vi "Cross-corelation.vi"() -> ()   [LabVIEW 2017]
uses:
  <vilib>/Analysis/1siggen.llb/General Gaussian Monopulse.vi
  <vilib>/Analysis/2dsp.llb/1D Cross Correlation (DBL).vi
  <vilib>/Analysis/NI_AALPro.lvlib
  <vilib>/Analysis/NI_AAL_SigProc.lvlib
  <vilib>/Analysis/NI_AALBase.lvlib
panel:
  in  "Number of samples to \nshift second signal":i32=11
  out "Waveforms":dbl[][](graph)
  out "Sample Delay":dbl
  out "Cross Corelation":dbl[](graph)
  # "Overview: This example uses cross correlation to determine the sample delay between two signals that are identical but have been shifted.\nRequirements: LabVIEW 2012 ( or compatible)\nInstructions: \n1. Input the configuration in the control\n2. Run the VI"
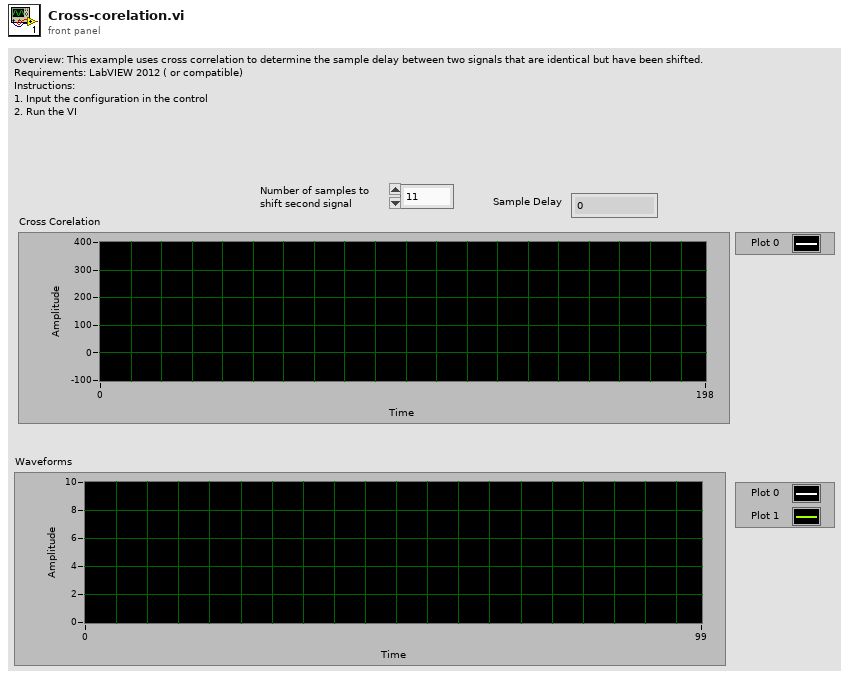
[diagram p1: front panel]
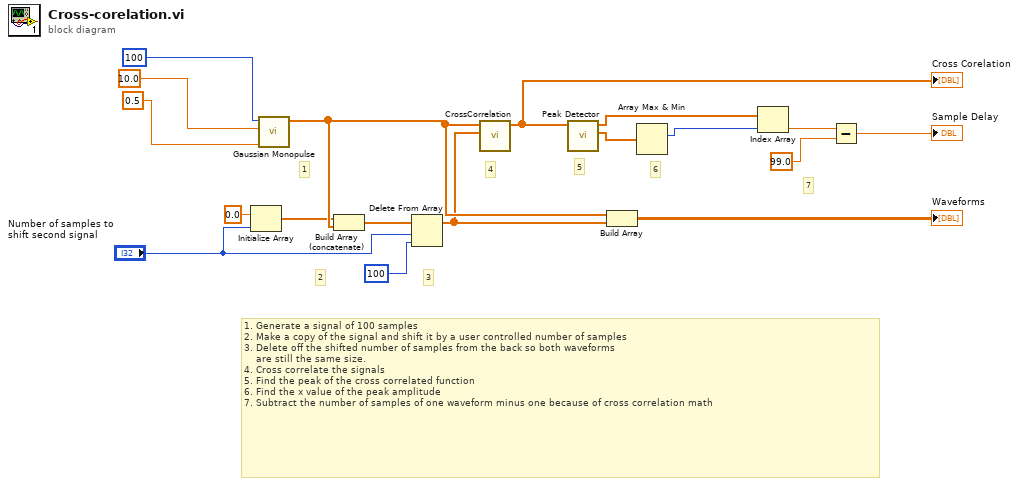
[diagram p0: block diagram]
diagram:
  # "7"
  # "6"
  # "5"
  # "4"
  # "3"
  # "2"
  # "1"
  # "1. Generate a signal of 100 samples\n2. Make a copy of the signal and shift it by a user controlled number of samples\n3. Delete off the shifted number of samples from the back so both waveforms\n    are still the same size.\n4. Cross correlate the signals\n5. Find the peak of the cross correlated function\n6. Find the x value of the peak amplitude\n7. Subtract the number of samples of one waveform minus one because of cross correlation math"
  n1 = Initialize Array(0.0 ("element"), "Number of samples to \nshift second signal") -> (w3:dbl[])
  n2 = call <vilib>:"Gaussian Monopulse.vi"("delta t (s)"=0.5 ("f2"), "amplitude"=10.0 ("f1"), "samples"=100) -> ("Gaussian Monopulse"=w5:dbl[])  [unwired: 7 in, 1 out]
  n3 = Build Array (concatenate)(w3, w5) -> (w7:dbl[])
  n4 = Delete From Array(array=w7, length="Number of samples to \nshift second signal", index=100) -> (array with subset deleted=w4:dbl[])  [unwired: 1 out]
  n5 = call-poly <vilib>:"CrossCorrelation.vi"("Y"=w4, "X"=w5) -> ("Rxy"=w18:dbl[])  [unwired: 8 in, 1 out]
  "Cross Corelation" <- w18
  n6 = call <vilib>:"Peak Detector.vi"("X"=w18) -> ("Amplitudes"=w17:dbl[], "Locations"=w15:dbl[])  [unwired: 6 in, 3 out]
  n7 = Build Array(w5, w4) -> (→"Waveforms":dbl[][])
  n8 = Array Max & Min(array=w17) -> (max index (indices)=w16:i32)  [unwired: 3 out]
  n9 = Index Array(array=w15, index=w16) -> (element=w14:dbl)
  n10 = Subtract(x=w14, y=99.0) -> (x-y=→"Sample Delay":dbl)
